vi "DataGraph_OutputData.vi"(9 "Data In":T1, 11 "Mass_Graph":refnum<vi>) -> ()   [LabVIEW 2018, in "DataGraphXControl.xctl"]
uses:
  DataGraphXControl.xctl
  DataGraph_Data.ctl
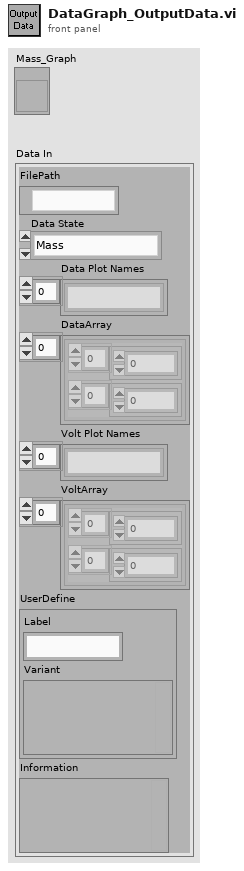
[diagram p1: front panel]
types:
  T1 = typedef "DataGraphXControl.xctl/DataGraph_Data.ctl" = cluster{"FilePath":path, "Data State":enum16{"Mass", "XIC"}, "Data Plot Names":string[], "DataArray":cluster{"X":dbl[], "Y":dbl[]}[], "Volt Plot Names":string[], "VoltArray":cluster{"X":dbl[], "Y":dbl[]}[], "UserDefine":cluster{"Label":string, "Variant":variant}, "Information":variant}
  T2 = enum16{"open", "replace", "create", "open or create", "replace or create", "replace or create with confirmation"}
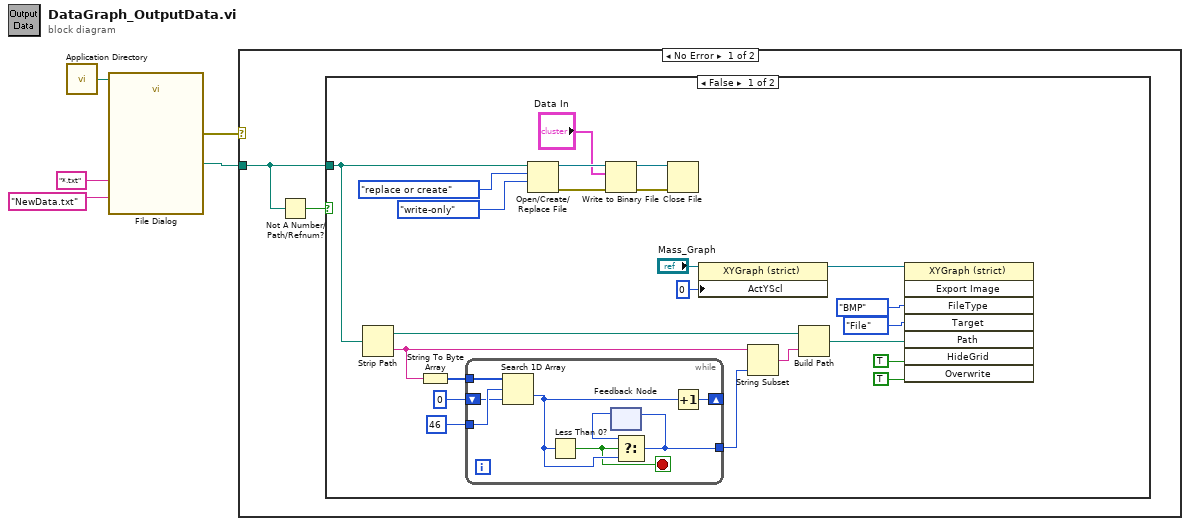
[diagram p0: block diagram]
diagram:
  n1 = call <vilib>:"Application Directory.vi"() -> ("Application Directory"=w4:path)
  n2 = call "File Dialog"("start path"=w4, "default name"="NewData.txt", "pattern (all files)"="*.txt") -> ("selected path"=w1:path, "error out"=w2:errorcluster)  [unwired: 9 in, 2 out]
  n3 = case shown="No Error" w2 {
    tunnel: w1 -> [w6 _]
    frame No Error {
      n4 = Not A Number/Path/Refnum?(number/path/refnum=w6) -> (NaN/Path/Refnum?=w7:bool)
      n5 = case shown="False" w7 {
        tunnel: w6 -> [w8 _]
        frame False {
          n6 = Strip Path(path=w8) -> (stripped path=w11:path, name=w12:string)
          n7 = String To Byte Array(string=w12) -> (unsigned byte array=w16:u8[])
          n8 = while {
            tunnel: w16 -> [w38]
            shift-right: [w36] -> _
            shift-left: 0 -> [w35]
            tunnel: u8 46 ("element") -> [w37]
            tunnel: [w32] -> w13
            stop <- w31 stop-if-true
            n9 = Search 1D Array(1D array=w38, element=w37, start index (0)=w35) -> (index of element=w33:i32)
            n10 = Less Than 0?(x=w33) -> (x < 0?=w31:bool)
            n11 = feedback #1() -> (w34:i32)  [unwired: 1 in]
            n12 = Select(t=w34, s=w31, f=w33) -> (s? t:f=w32:i32)
            n13 = feedback-in #1(w32) -> ()
            n14 = Increment(x=w33) -> (x+1=w36:i32)
          }
          n15 = Open/Create/Replace File(file path (use dialog)=w8, operation (0:open)=T2."replace or create", access (0:read/write)=enum16{"read/write", "read-only", "write-only"}."write-only") -> (refnum out=w30:refnum<file>, error out=w28:errorcluster)  [unwired: 3 in, 1 out]
          n16 = Write to Binary File(file (use dialog)=w30, data="Data In", error in=w28) -> (refnum out=w29:refnum<file>, error out=w27:errorcluster)  [unwired: 3 in, 1 out]
          n17 = Close File(refnum=w29, error in=w27) -> ()  [unwired: 2 out]
          n18 = property class="XYGraph (strict)"(reference="Mass_Graph", "ActYScl"=0 ("Active Y Scale")) -> (reference out=w18:refnum<vi>)  [unwired: 1 in, 1 out]
          n19 = String Subset(string=w12, length (rest)=w13) -> (substring=w10:string)  [unwired: 1 in]
          n20 = Build Path(base path=w11, name or relative path=w10) -> (appended path=w9:path)
          n21 = invoke class="XYGraph (strict)" method="Export Image"(reference=w18, "FileType"=enum32{"BMP", "EPS", "EMF", "PICT"}."BMP" ("File Type"), "Target"=enum32{"File", "Clipboard"}."File", "Path"=w9, "HideGrid"=TRUE ("Hide Grid"), "Overwrite"=TRUE ("Always Overwrite")) -> ()  [unwired: 2 in, 8 out]
        }
        frame True {
        }
      }
    }
    frame Error {
    }
  }
